vi "Clear Charact Results.vi"(11 "error in":errorcluster) -> (15 "error out":errorcluster)   [LabVIEW 2023, in "RFFixtureCharact.Public.lvlib"]
uses:
  RFFixtureCharact.Public.lvlib
  Type Definitions/Collection Operation.ctl
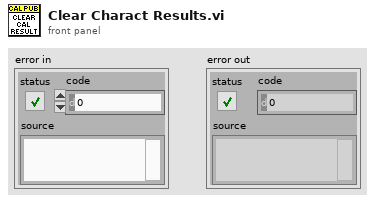
[diagram p1: front panel]
types:
  T1 = typedef "RFFixtureCharact.Public.lvlib/Collection Operation.ctl" = enum16{"Append", "Get", "Get All", "Clear"}
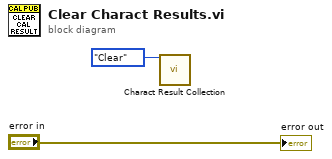
[diagram p0: block diagram]
diagram:
  n1 = call "Charact Result Collection.vi"("Operation"=Collection_Operation."Clear") -> ()  [unwired: 13 in, 2 out]
  "error out" <- "error in"
